vi "New Main Log Loop.vi"(8 "error in (no error)":errorcluster) -> (0 "error out":errorcluster)   [LabVIEW 2015]
uses:
  Packet Types.ctl
  Robot Global Data.vi
panel:
  out "result string":string
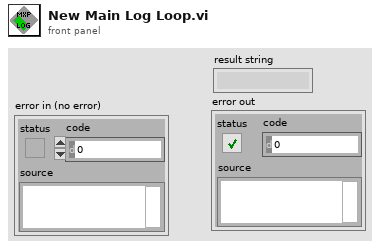
[diagram p1: front panel]
types:
  T1 = typedef "packet types.ctl" = enum16{"Log line", "Open File", "Send Header", "Set Time", "Send to LCD"}
  T2 = typedef "Packet Types.ctl" = enum16{"Log line", "Open File", "Send Header", "Set Time", "Send to LCD"}
  T3 = typedef "WPI_SerialPortRef.ctl" = cluster{"DevStatus":errorcluster, "Serial Port Name":refnum<visa-resource-name>}
  T4 = typedef "WPI_DriverStationRobotMode2.ctl" = enum16{"Autonomous Disabled", "Autonomous Enabled", "Teleop Disabled", "Teleop Enabled", "Disconnected", "Finish", "Test Disabled", "Test Enabled", "Emergency Stopped"}
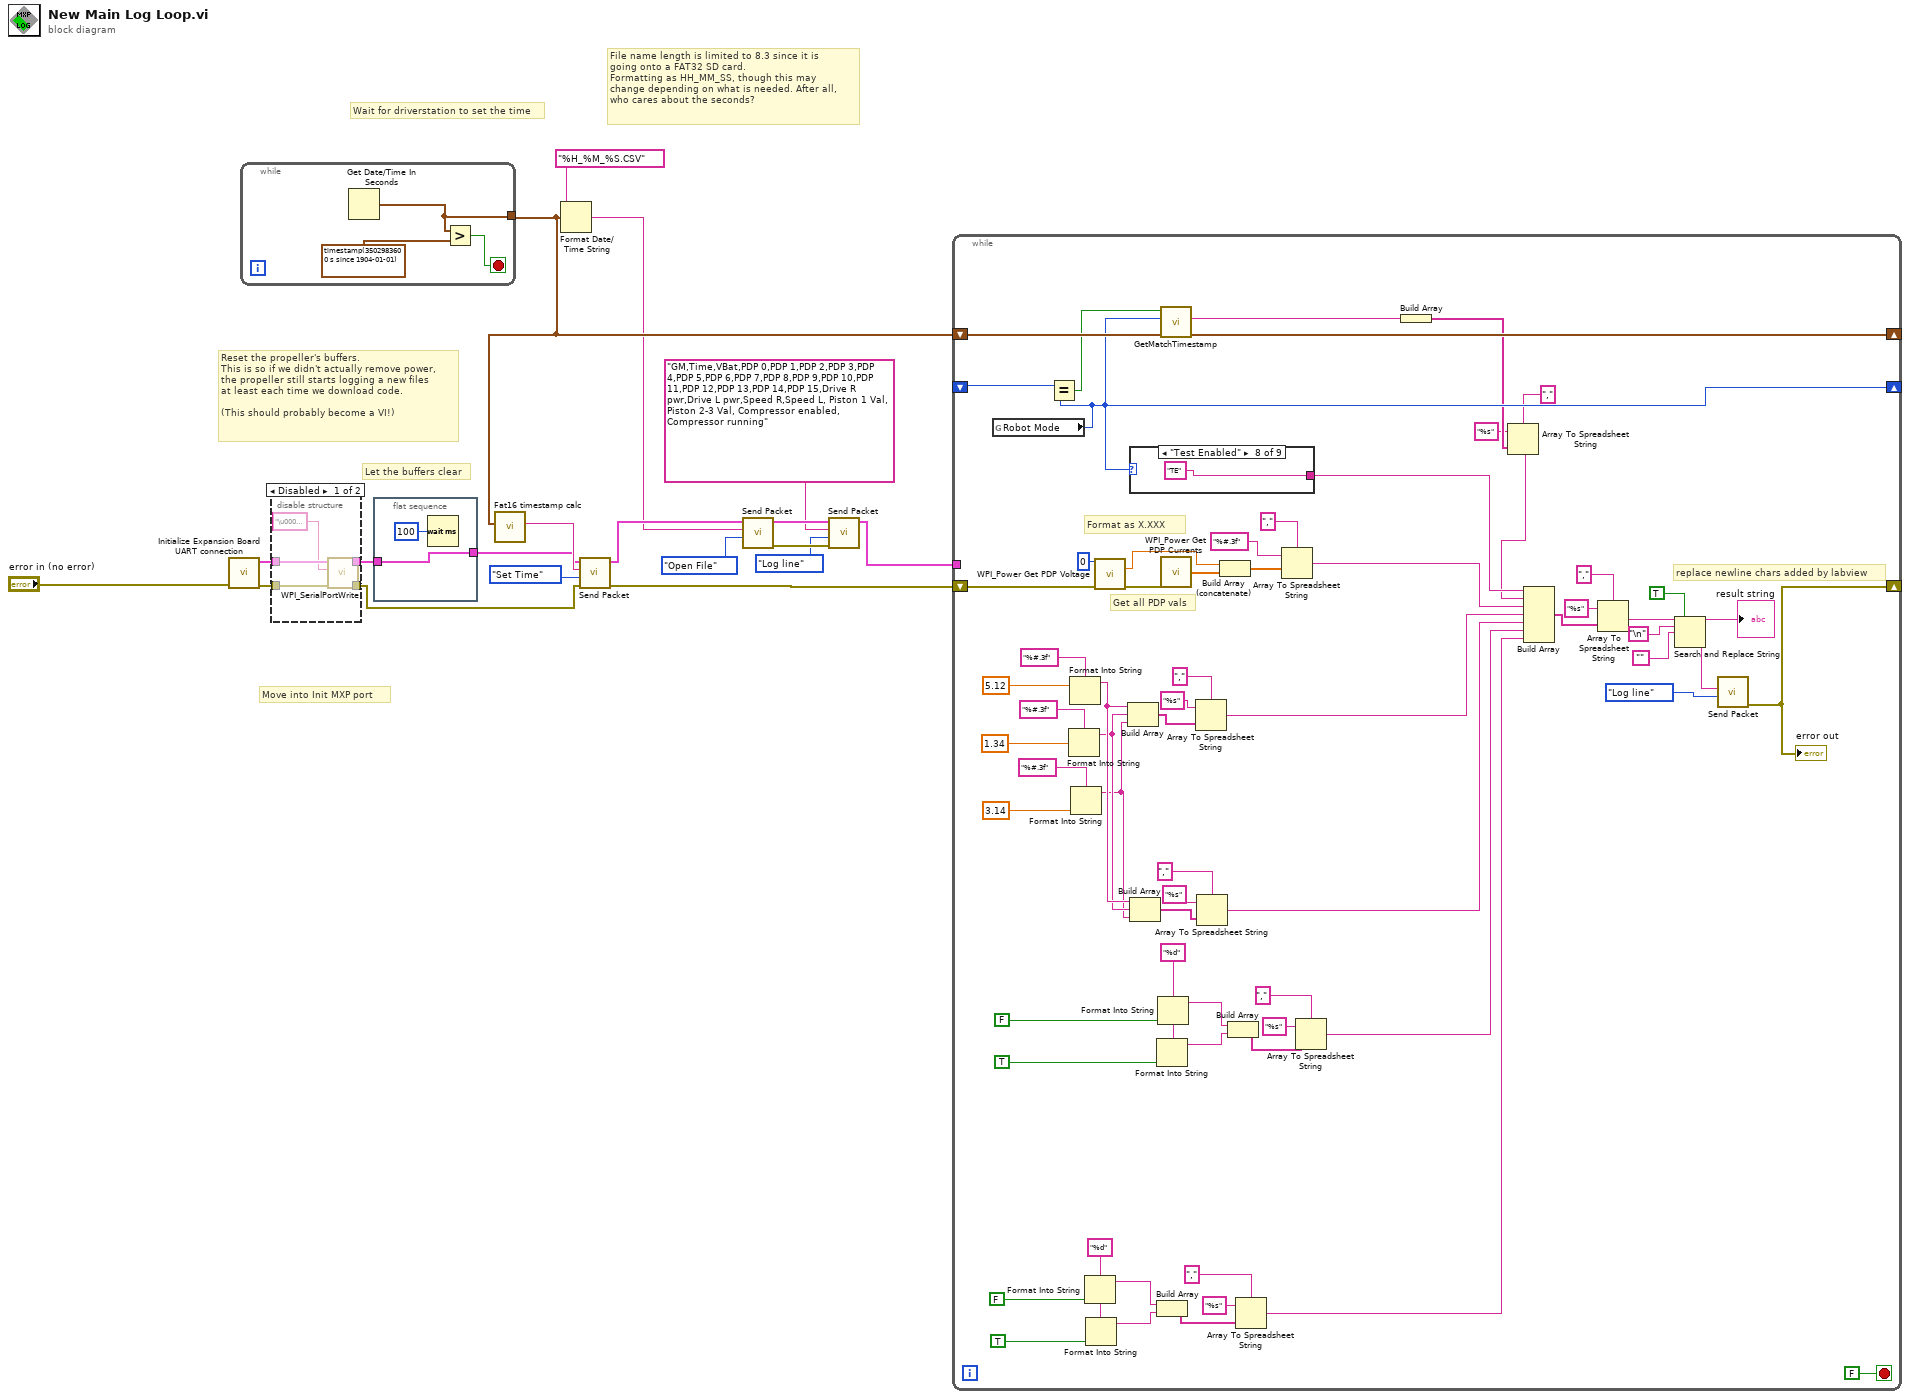
[diagram p0: block diagram]
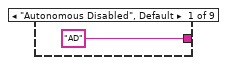
[diagram p2: hidden frame]
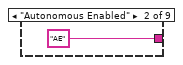
[diagram p3: hidden frame]
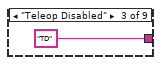
[diagram p4: hidden frame]
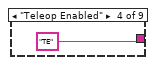
[diagram p5: hidden frame]
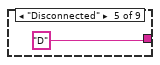
[diagram p6: hidden frame]
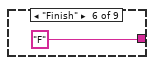
[diagram p7: hidden frame]
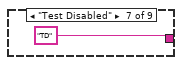
[diagram p8: hidden frame]
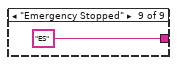
[diagram p9: hidden frame]
diagram:
  # "Move into Init MXP port"
  # "Let the buffers clear"
  # "Reset the propeller's buffers.\nThis is so if we didn't actually remove power,\nthe propeller still starts logging a new files \nat least each time we download code.\n\n(This should probably become a VI!)"
  # "File name length is limited to 8.3 since it is \ngoing onto a FAT32 SD card. \nFormatting as HH_MM_SS, though this may\nchange depending on what is needed. After all,\nwho cares about the seconds?"
  # "Wait for driverstation to set the time"
  n1 = call "Initialize Expansion Board UART connection.vi"("error in (no error)"="error in (no error)") -> ("error out"=w16:errorcluster, "SerialPortRef"=w15:T3)  [unwired: 9 in]
  n2 = while {
    tunnel: [w20] -> w10
    stop <- w21 stop-if-true
    n3 = Get Date/Time In Seconds() -> (seconds since 1Jan1904=w20:timestamp)
    n4 = Greater?(x=w20, y=timestamp(3502983600 s since 1904-01-01)) -> (0:w21:bool)
  }
  n5 = disable-structure shown="Disabled" {
    disable-tunnel: w16 -> [w27 w28]
    disable-tunnel: w15 -> [w26 w29]
    disable-tunnel: [w24 w29] -> w13
    disable-tunnel: [w23 w28] -> w12
    frame Disabled {
      n6 = call <vilib>:"WPI_SerialPortWrite.vi"("error in (no error)"=w27, "Buffer"="\u0004\u0004", "SerialPortRef"=w26) -> ("error out"=w23:errorcluster, "SerialPortRef"=w24:T3)  [unwired: 6 in, 1 out]
    }
    frame Enabled {
    }
  }
  n7 = flat-sequence {
    tunnel: [w31] -> w14
    tunnel: w13 -> [w31]
    frame #0 {
      n8 = Wait (ms)(milliseconds to wait=u32 100) -> ()  [unwired: 1 out]
    }
  }
  n9 = call "Fat16 timestamp calc.vi"("time stamp"=w10) -> ("timestamp as string"=w18:string)  [unwired: 10 in]
  n10 = Format Date/Time String(time format string (%c)="%H_%M_%S.CSV", seconds (now)=w10) -> (date/time string=w3:string)  [unwired: 1 in]
  n11 = call "Send Packet.vi"("error in (no error)"=w12, 7:Packet_Types."Set Time", "Log string"=w18, "SerialPortRef"=w14) -> ("error out"=w1:errorcluster, "SerialPortRef out"=w4:T3)  [unwired: 4 in]
  n12 = call "Send Packet.vi"(7:packet_types."Open File", "Log string"=w3, "SerialPortRef"=w4) -> ("error out"=w8:errorcluster, "SerialPortRef out"=w9:T3)  [unwired: 5 in]
  n13 = call "Send Packet.vi"("error in (no error)"=w8, 7:packet_types."Log line", "Log string"="GM,Time,VBat,PDP 0,PDP 1,PDP 2,PDP 3,PDP 4,PDP 5,PDP 6,PDP 7,PDP 8,PDP 9,PDP 10,PDP 11,PDP 12,PDP 13,PDP 14,PDP 15,Drive R pwr,Drive L pwr,Speed R,Speed L, Piston 1 Val, Piston 2-3 Val, Compressor enabled, Compressor running", "SerialPortRef"=w9) -> ("SerialPortRef out"=w5:T3)  [unwired: 4 in, 1 out]
  n14 = while {
    shift-right: [w97] -> _
    shift-left: w10 -> [w96]
    shift-right: [w93] -> _
    shift-left: _ -> [w95]
    tunnel: w5 -> [_]
    shift-right: [w64] -> _
    shift-left: w1 -> [w63]
    stop <- FALSE stop-if-true
    w47 = "%d" ("format string")
    w48 = "%d" ("format string")
    # "Get all PDP vals"
    # "replace newline chars added by labview"
    # "Format as X.XXX"
    n15 = global read "Robot Global Data.vi" "Robot Mode"() -> (w93:T4)
    n16 = Equal?(x=w95, y=w93) -> (x = y?=w94:bool)
    n17 = Format Into String(format string="%#.3f", 1.34 ("input 1")) -> (resulting string=w36:string)  [unwired: 2 in, 1 out]
    n18 = Format Into String(format string="%#.3f", 5.12 ("input 1")) -> (resulting string=w37:string)  [unwired: 2 in, 1 out]
    n19 = Format Into String(format string="%#.3f", 3.14 ("input 1")) -> (resulting string=w35:string)  [unwired: 2 in, 1 out]
    n20 = Format Into String(format string=w47, FALSE ("input 1")) -> (resulting string=w61:string)  [unwired: 2 in, 1 out]
    n21 = Format Into String(format string=w47, TRUE ("input 1")) -> (resulting string=w60:string)  [unwired: 2 in, 1 out]
    n22 = call <vilib>:"WPI_Power Get PDP Voltage.vi"("Power Distribution Panel (0)"=u8 0, "error in"=w63) -> ("voltage (V)"=w87:dbl, "error out"=w84:errorcluster)  [unwired: 12 in]
    n23 = Build Array(w37, w36, w35) -> (w43:string[])
    n24 = case shown="\"Test Enabled\"" w93 {
      tunnel: ["AD" "AE" "TD" "TE" "D" "F" "TD" "TE" "ES"] -> w92
      frame "Autonomous Disabled", Default {
      }
      frame "Autonomous Enabled" {
      }
      frame "Teleop Disabled" {
      }
      frame "Teleop Enabled" {
      }
      frame "Disconnected" {
      }
      frame "Finish" {
      }
      frame "Test Disabled" {
      }
      frame "Test Enabled" {
      }
      frame "Emergency Stopped" {
      }
    }
    n25 = Build Array(w37, w36, w35) -> (w32:string[])
    n26 = Format Into String(format string=w48, TRUE ("input 1")) -> (resulting string=w75:string)  [unwired: 2 in, 1 out]
    n27 = Build Array(w61, w60) -> (w62:string[])
    n28 = Format Into String(format string=w48, FALSE ("input 1")) -> (resulting string=w76:string)  [unwired: 2 in, 1 out]
    n29 = call "GetMatchTimestamp.vi"("seconds since 1Jan1904"=w96, "Robot Mode"=w93, "Boolean"=w94) -> ("seconds since 1Jan1904 2"=w97:timestamp, "Match Timestamp"=w53:string)  [unwired: 7 in]
    n30 = call <vilib>:"WPI_Power Get PDP Currents.vi"("error in"=w84) -> ("all currents (A)"=w85:dbl[])  [unwired: 12 in, 2 out]
    n31 = Array To Spreadsheet String(delimiter (Tab)=",", array=w43, 3:"%s" ("format string")) -> (spreadsheet string=w78:string)
    n32 = Array To Spreadsheet String(delimiter (Tab)=",", array=w32, 3:"%s" ("format string")) -> (spreadsheet string=w79:string)
    n33 = Build Array (concatenate)(w87, w85) -> (w86:dbl[])
    n34 = Build Array(w76, w75) -> (w77:string[])
    n35 = Array To Spreadsheet String(delimiter (Tab)=",", array=w62, 3:"%s" ("format string")) -> (spreadsheet string=w51:string)
    n36 = Array To Spreadsheet String(delimiter (Tab)=",", array=w86, 3:"%#.3f" ("format string")) -> (spreadsheet string=w83:string)
    n37 = Array To Spreadsheet String(delimiter (Tab)=",", array=w77, 3:"%s" ("format string")) -> (spreadsheet string=w73:string)
    n38 = Build Array(w53) -> (w52:string[])
    n39 = Array To Spreadsheet String(delimiter (Tab)=",", array=w52, 3:"%s" ("format string")) -> (spreadsheet string=w82:string)
    n40 = Build Array(w92, w82, w83, w78, w79, w73, w51) -> (w67:string[])
    n41 = Array To Spreadsheet String(delimiter (Tab)=",", array=w67, 3:"%s" ("format string")) -> (spreadsheet string=w68:string)
    n42 = Search and Replace String(replace all?=TRUE ("replace all? (F)"), input string=w68, search string="\n", replace string="") -> (result string=w66:string)  [unwired: 4 in, 3 out]
    "result string" <- w66
    n43 = call "Send Packet.vi"(7:packet_types."Log line", "Log string"=w66) -> ("error out"=w64:errorcluster)  [unwired: 6 in, 1 out]
    "error out" <- w64
  }
